vi "dfd_Render ZPK Gain.vi"(5 "Fonts Input":T3(array[cluster]), 7 "format coeffiecients":string="%#g", 8 "gain":dbl, 9 "alignment(left, top)":T2, 10 "origin":cluster{"x":i16, "y":i16}, 11 "picture in":picture) -> (2 "text rect":T1, 3 "picture out":picture)   [LabVIEW 2017, in "NI_DigFilter_Process.lvlib"]
uses:
  <vilib>/addons/Digital Filter Design/NI_DigFilter_Process.lvlib
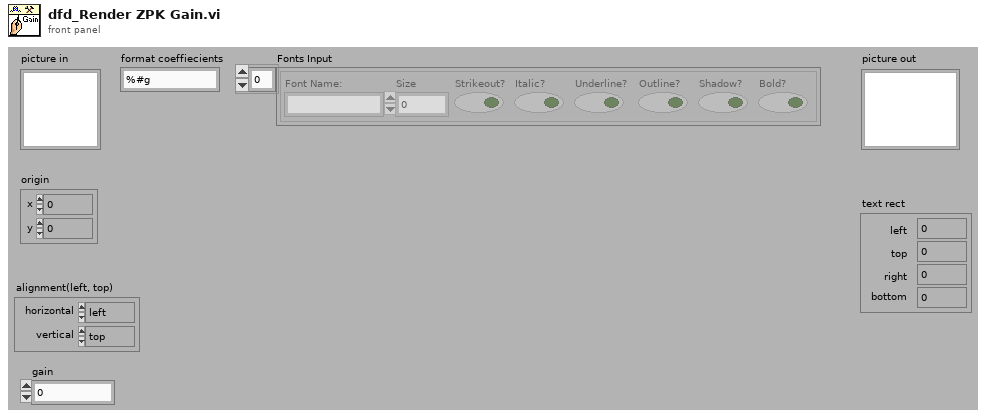
[diagram p1: front panel]
types:
  T1 = cluster{"left":i16, "top":i16, "right":i16, "bottom":i16}
  T2 = cluster{"horizontal":enum16{"left", "center", "right"}, "vertical":enum16{"top", "center", "bottom"}}
  T3 = cluster{"Font Name:":string, "Size":i16, "Strikeout?":bool, "Italic?":bool, "Underline?":bool, "Outline?":bool, "Shadow?":bool, "Bold?":bool}[]
  T4 = enum16{"User-specified Font", "Application Font", "System Font", "Dialog Font"}
  T5 = cluster{"Font Name:":string, "Size":i16, "Strikeout?":bool, "Italic?":bool, "Underline?":bool, "Outline?":bool, "Shadow?":bool, "Bold?":bool}
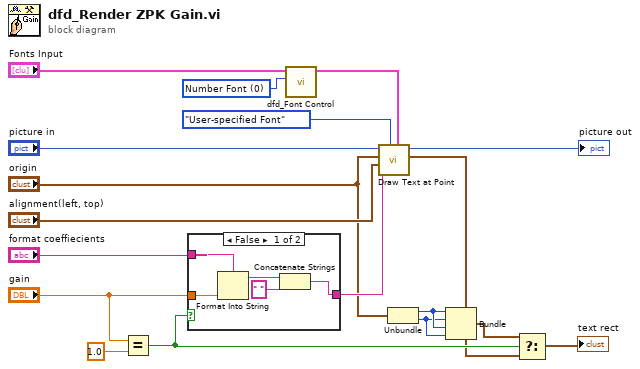
[diagram p0: block diagram]
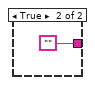
[diagram p2: hidden frame]
diagram:
  w16 = u16 0 items=["Number Font", "Variable Font", "Script Font"] ("Tpye")
  n1 = Equal?(x="gain", y=1.0 ("x")) -> (x = y?=w6:bool)
  n2 = case shown="False" w6 {
    tunnel: "gain" -> [w23 _]
    tunnel: "format coeffiecients" -> [w21 _]
    tunnel: [w20 ""] -> w11
    frame False {
      n3 = Format Into String(format string=w21, w23) -> (resulting string=w22:string)  [unwired: 2 in, 1 out]
      n4 = Concatenate Strings(w22, " ") -> (w20:string)
    }
    frame True {
    }
  }
  n5 = call <vilib>:"dfd_Font Control.vi"("tpye"=w16, "fonts input"="Fonts Input") -> ("font output"=w14:T5)  [unwired: 9 out]
  n6 = call <vilib>:"Draw Text at Point.vi"("[user-specified font]"=w14, "desired font(Application)"=T4."User-specified Font", "text"=w11, "alignment(left, top)"="alignment(left, top)", "origin"="origin", "picture"="picture in") -> ("text rect"=w1:T1, "new picture"=→"picture out":picture)  [unwired: 3 in, 1 out]
  n7 = Unbundle("origin") -> ("x"=w7:i16, "y"=w2:i16)
  n8 = Bundle(cluster=w1, "left"=w7, "top"=w2, "right"=w7, "bottom"=w2) -> (w4:T1)
  n9 = Select(t=w4, s=w6, f=w1) -> (s? t:f=→"text rect":T1)
